vi "Create.vi"(5 "Coverage in":refnum<class "Coverage.lvclass">, 8 "error in (no error)":errorcluster, 11 "Timestamp":timestamp) -> (0 "error out":errorcluster, 3 "Coverage":refnum<class "Coverage.lvclass">)   [LabVIEW 2017, in "Cobertura.lvlib" / "Coverage.lvclass"]
uses:
  Coverage.lvclass
  Coverage.lvclass/Coverage.ctl
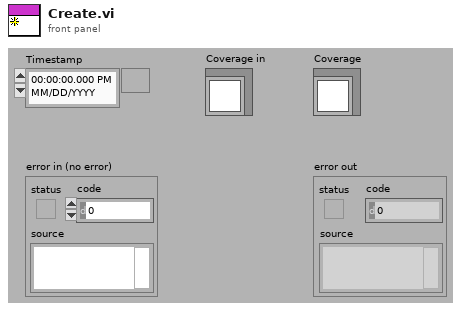
[diagram p1: front panel]
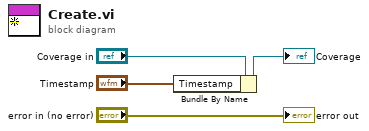
[diagram p0: block diagram]
diagram:
  n1 = Bundle By Name(cluster="Coverage in", "Timestamp"="Timestamp") -> (→"Coverage":refnum<class "Coverage.lvclass">)
  "error out" <- "error in (no error)"
